vi "StepperMove.vi"(8 "error in":errorcluster) -> ()   [LabVIEW 2015]
doc: "Commands\n 0 - set units (0-inHg, 1-mmHg, 2-torr, 3-mbar)\n 1 - set vacuum zero\n 2 - reserved\n 3 - reserved\n 4 - reserved\n 5 - set vacuum calibration\n 6 - reserved\n 7 - start bootloader\n 8 - get firmware version\n 9 - get vacuum reading\n 10 - start/stop vacuum control (0-stop, 1-start)\n 11 - set vacuum setpoint\n 12 - set calibration zero offset (prevent negative zero value from DWIN)\n 13 - set pump speed 0-100 \n 14 - set vacuum valve PWM 0-1000\n 15 - set bleed valve PWM 0-1000"
panel:
  out "element":string
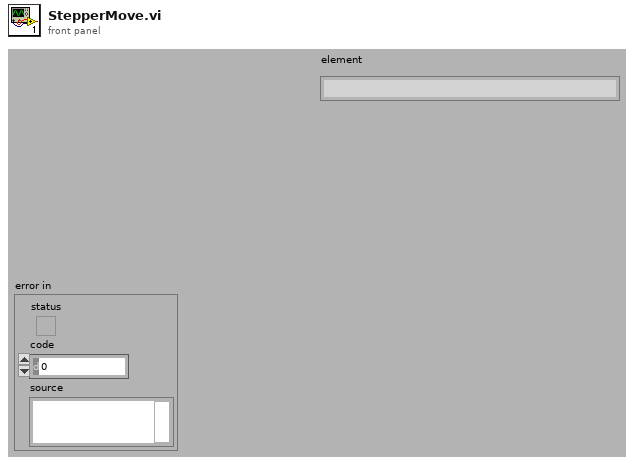
[diagram p1: front panel]
types:
  T1 = enum16{"usbSetEnable", "usbSetDirection", "usbSetCounts", "usbSetClock", "usbStartMotion"}
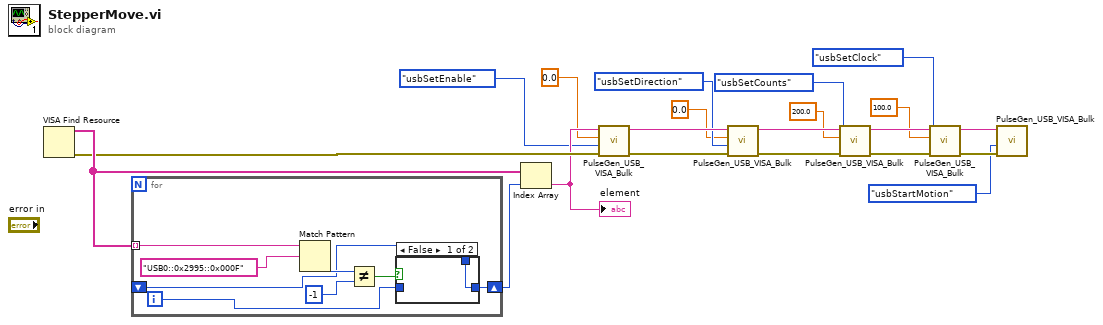
[diagram p0: block diagram]
diagram:
  n1 = VISA Find Resource() -> (0:w19:errorcluster, 3:w21:string[])  [unwired: 3 in, 1 out]
  n2 = for {
    tunnel: w21 -> [w29] mode=indexing
    shift-right: [w23] -> w20
    shift-left: _ -> [w22]
    i -> [w24]
    n3 = Match Pattern(string=w29, regular expression="USB0::0x2995::0x000F" ("element")) -> (offset past match=w27:i32)  [unwired: 1 in, 3 out]
    n4 = Not Equal?(x=w27, y=-1) -> (x != y?=w25:bool)
    n5 = case shown="False" w25 {
      tunnel: w24 -> [_ w31]
      tunnel: [w30 w31] -> w23
      tunnel: w22 -> [w30 _]
      frame False {
      }
      frame True {
      }
    }
  }
  n6 = Index Array(array=w21, index=w20) -> (element=w18:string)
  "element" <- w18
  n7 = call "PulseGen_USB_VISA_Bulk.vi"("error in"=w19, "Command Index"=T1."usbSetEnable", "Numeric Input (Optional)"=sgl 0.0, "Resource Name"=w18) -> ("error out"=w15:errorcluster, "Resource Name 2"=w14:string)  [unwired: 5 in, 1 out]
  n8 = call "PulseGen_USB_VISA_Bulk.vi"("error in"=w15, "Command Index"=T1."usbSetDirection", "Numeric Input (Optional)"=sgl 0.0, "Resource Name"=w14) -> ("error out"=w11:errorcluster, "Resource Name 2"=w10:string)  [unwired: 5 in, 1 out]
  n9 = call "PulseGen_USB_VISA_Bulk.vi"("error in"=w11, "Command Index"=T1."usbSetCounts", "Numeric Input (Optional)"=sgl 200.0, "Resource Name"=w10) -> ("error out"=w7:errorcluster, "Resource Name 2"=w6:string)  [unwired: 5 in, 1 out]
  n10 = call "PulseGen_USB_VISA_Bulk.vi"("error in"=w7, "Command Index"=T1."usbSetClock", "Numeric Input (Optional)"=sgl 100.0, "Resource Name"=w6) -> ("error out"=w3:errorcluster, "Resource Name 2"=w2:string)  [unwired: 5 in, 1 out]
  n11 = call "PulseGen_USB_VISA_Bulk.vi"("error in"=w3, "Command Index"=T1."usbStartMotion", "Resource Name"=w2) -> ()  [unwired: 6 in, 3 out]
